vi "GetButtonModel.vi"(8 "error in (no error)":errorcluster caption="错误输入（无错误）", 11 "按键型号":refnum<vi>) -> (0 "error out":errorcluster caption="错误输出")   [LabVIEW 2013]
uses:
  GlobalValue.vi
  <vilib>/Utility/config.llb/NI_LVConfig.lvlib
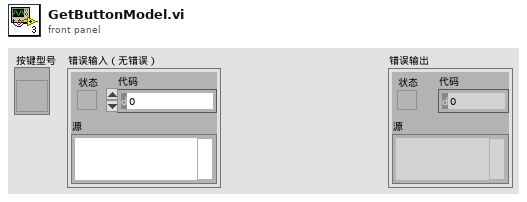
[diagram p1: front panel]
types:
  T1 = typedef "NI_LVConfig.lvlib/Config Data RefNum.ctl" = refnum<k1>
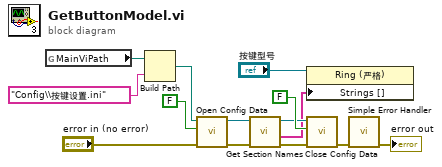
[diagram p0: block diagram]
diagram:
  n1 = global read "GlobalValue.vi" "MainViPath"() -> (w1:path)
  n2 = Build Path(base path=w1, name or relative path="Config\\按键设置.ini" ("名称或相对路径")) -> (appended path=w11:path)
  n3 = call <vilib>:"Open Config Data.vi"("error in (no error)"="error in (no error)", "create file if necessary (T)"=FALSE ("create file if necessary? (T)"), "configuration file path"=w11) -> ("error out"=w8:errorcluster, "refnum"=w9:T1)  [unwired: 6 in, 1 out]
  n4 = call <vilib>:"Get Section Names.vi"("error in (no error)"=w8, "refnum"=w9) -> ("error out"=w7:errorcluster, "section names"=w4:string[], "refnum out"=w6:T1)  [unwired: 7 in]
  n5 = property on="属性节点" class="Ring (严格)"(reference="按键型号", "Strings []"=w4) -> ()  [unwired: 1 in, 2 out]
  n6 = call <vilib>:"Close Config Data.vi"("error in (no error)"=w7, "write file if changed (T)"=FALSE ("write configuration file? (T)"), "refnum"=w6) -> ("error out"=w12:errorcluster)  [unwired: 8 out]
  n7 = call <vilib>:"Simple Error Handler.vi"("error in (no error)"=w12) -> ("error out"=→"error out":errorcluster)  [unwired: 1 in, 7 out]
